vi "LDF Get Sch Name.vi"(9 "pSchName":string, 10 "index":i32, 11 "LDFHandle":u64) -> (1 "pSchName out":string, 3 "function return":i32)   [LabVIEW 2010, in "ldf_parser.lvlib"]
doc: "int WINAPI LDF_GetSchName(long long LDFHandle, int index, char* pSchName);"
uses:
  ldf_parser.lvlib
  USB2XXX/trunk/USB2XXX/USB2XXX/vs2019/Release/USB2XXX.dll
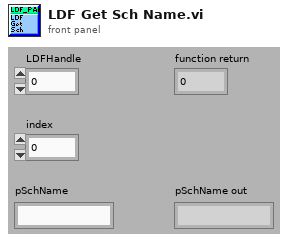
[diagram p1: front panel]
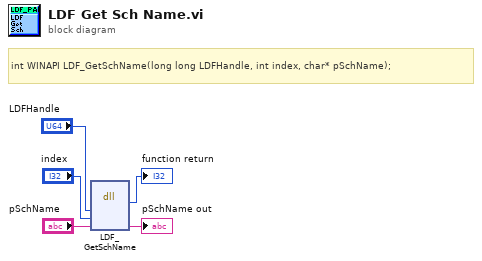
[diagram p0: block diagram]
diagram:
  # "int WINAPI LDF_GetSchName(long long LDFHandle, int index, char* pSchName);"
  n1 = dll-call lib="E:/Projects/USB2XXX/trunk/USB2XXX/USB2XXX/vs2019/Release/USB2XXX.*" fn="LDF_GetSchName"("LDFHandle"="LDFHandle", "index"="index", "pSchName"="pSchName") -> (→"function return":i32, "pSchName"=→"pSchName out":string)  [unwired: 5 in, 2 out]
